vi "analogO.vi"() -> ()   [LabVIEW 2016]
panel:
  in  "Amplitude":dbl=1.0
  in  "Frequency":dbl=10.1
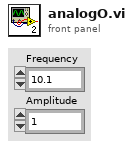
[diagram p1: front panel]
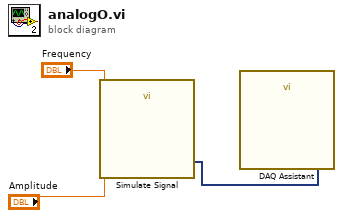
[diagram p0: block diagram]
diagram:
  n1 = call "Simulate Signal"("Frequency"="Frequency", "Amplitude"="Amplitude") -> ("Sawtooth"=w1:dynamicdata)  [unwired: 12 in, 1 out]
  n2 = call "DAQ Assistant"("data"=w1) -> ()  [unwired: 17 in, 2 out]
